vi "autonomous hard code.vi"   [LabVIEW 2012]
uses:
  <vilib>/Rock Robotics/WPI/Solenoid/WPI_SolenoidValue.ctl
  <vilib>/Rock Robotics/WPI/Solenoid/WPI_SolenoidSetEnum.vi
types:
  T1 = typedef "WPI_SolenoidValue.ctl" = enum16{"Off", "On", "Forward", "Reverse"}
  T2 = typedef "WPI_MotorControlDeviceRef.ctl" = cluster{"DeviceStatus":errorcluster, "Type":enum16{"PWM", "CAN"}, "PWM":cluster{"Digital Module":T3, "PWM Channel":T4, "DeadBand":T5}, "CAN":cluster{"Device Number":u8, "Control Mode":T6, "Semaphore":T7, "Max Vout":dbl}, "Invert":bool, "TransformRef":T8, "InvTransformRef":T8}
  T3 = typedef "FPGA_TypedefDigitalModule.ctl" = enum16{"Digital Module 1", "Digital Module 2"}
  T4 = typedef "FPGA_DIOPWMChannel.ctl" = enum8{"PWM 1", "PWM 2", "PWM 3", "PWM 4", "PWM 5", "PWM 6", "PWM 7", "PWM 8", "PWM 9", "PWM 10", "Invalid"}
  T5 = typedef "WPI_PWMDeadband.ctl" = cluster{"Name":string, "maxPositivePwm":i32, "minPositivePwm":i32, "centerPwm":i32, "maxNegativePwm":i32, "minNegativePwm":i32, "angularRange":u16}
  T6 = typedef "WPI_CANJaguar_ControlMode.ctl" = enum8{"Percent VBus", "Current", "Speed", "Position", "Voltage"}
  T7 = typedef "Semaphore RefNum" = refnum<k1>
  T8 = typedef "WPI_PWMTransform_ConPane.ctl" = refnum<vi>
  T9 = typedef "WPI_AnalogChannelDevRef.ctl" = cluster{"DevStatus":errorcluster, "Analog Module":T10, "Analog Channel":T11}
  T10 = typedef "FPGA_TypedefAnalogModule.ctl" = enum16{"Analog Module 1", "Analog Module 2"}
  T11 = typedef "FPGA_AIChannel.ctl" = enum8{"AI 1", "AI 2", "AI 3", "AI 4", "AI 5", "AI 6", "AI 7", "AI 8", "Invalid"}
  T12 = typedef "WPI_SolenoidDevRef.ctl" = cluster{"DevStatus":errorcluster, "Solenoid Module":T13, "Forward Solenoid Channel":T14, "Reverse Solenoid Channel":T14}
  T13 = typedef "FPGA_TypedefSolenoidModule.ctl" = enum16{"Solenoid Module 1", "Solenoid Module 2"}
  T14 = typedef "WPI_SolenoidChannel.ctl" = enum8{"Solenoid 1", "Solenoid 2", "Solenoid 3", "Solenoid 4", "Solenoid 5", "Solenoid 6", "Solenoid 7", "Solenoid 8", "Invalid"}
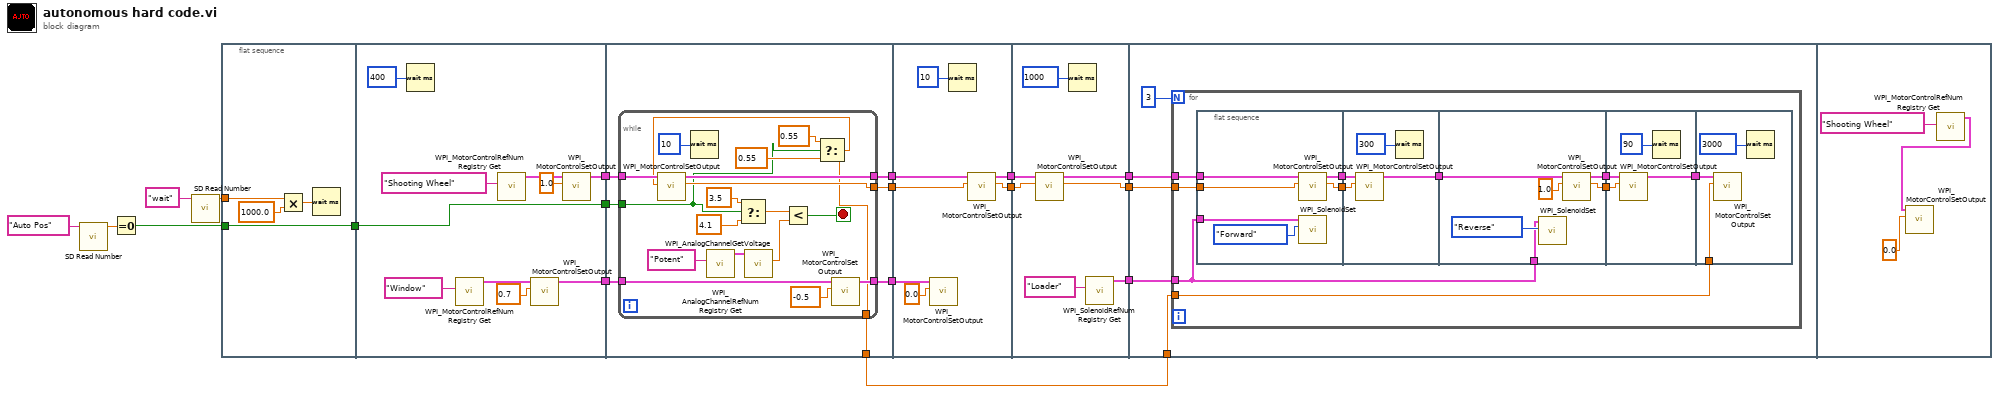
[diagram p0: block diagram]
diagram:
  n1 = call <vilib>:"SD Read Number.vi"("Name"="Auto Pos") -> ("Numeric"=w18:dbl)  [unwired: 8 in, 2 out]
  n2 = Equal To 0?(x=w18) -> (x = 0?=w14:bool)
  n3 = call <vilib>:"SD Read Number.vi"("Name"="wait") -> ("Numeric"=w15:dbl)  [unwired: 8 in, 2 out]
  n4 = flat-sequence {
    tunnel: w15 -> [w21]
    tunnel: [w19] -> w13
    tunnel: w14 -> [w19]
    tunnel: w13 -> [w27]
    tunnel: [w27] -> w12
    tunnel: [w29] -> w11
    tunnel: [w24] -> w6
    tunnel: w12 -> [w38]
    tunnel: w11 -> [w39]
    tunnel: [w37] -> w10
    tunnel: [w36] -> w9
    tunnel: w6 -> [w35]
    tunnel: [w34] -> w5
    tunnel: [w33] -> w1
    tunnel: w10 -> [w63]
    tunnel: w9 -> [w61]
    tunnel: [w60] -> w8
    tunnel: w5 -> [w59]
    tunnel: [w58] -> w4
    tunnel: w8 -> [w71]
    tunnel: [w69] -> w7
    tunnel: w4 -> [w68]
    tunnel: [w67] -> w3
    tunnel: [w65] -> w2
    tunnel: w7 -> [w76]
    tunnel: w3 -> [w72]
    tunnel: w1 -> [w75]
    tunnel: w2 -> [w73]
    frame #0 {
      n5 = Multiply(x=w21, y=1000.0) -> (x*y=w20:dbl)
      n6 = Wait (ms)(milliseconds to wait=w20) -> ()  [unwired: 1 out]
    }
    frame #1 {
      n7 = Wait (ms)(milliseconds to wait=u32 400) -> ()  [unwired: 1 out]
      n8 = call <vilib>:"WPI_MotorControlRefNum Registry Get.vi"("refnum name"="Window") -> ("MotorControlDevRef"=w32:T2)  [unwired: 9 in, 1 out]
      n9 = call <vilib>:"WPI_MotorControlRefNum Registry Get.vi"("refnum name"="Shooting Wheel") -> ("MotorControlDevRef"=w25:T2)  [unwired: 9 in, 1 out]
      n10 = call <vilib>:"WPI_MotorControlSetOutput.vi"("Output"=0.7, "MotorControlDevRef"=w32) -> ("MotorControlDevRef"=w29:T2)  [unwired: 7 in, 2 out]
      n11 = call <vilib>:"WPI_MotorControlSetOutput.vi"("Output"=1.0, "MotorControlDevRef"=w25) -> ("MotorControlDevRef"=w24:T2)  [unwired: 7 in, 2 out]
    }
    frame #2 {
      n12 = while {
        tunnel: w39 -> [w57]
        tunnel: w38 -> [w42]
        tunnel: [w48] -> w37
        tunnel: [w47] -> w36
        tunnel: w35 -> [w46]
        tunnel: [w45] -> w34
        tunnel: [w40] -> w33
        stop <- w50 stop-if-true
        n13 = Wait (ms)(milliseconds to wait=u32 10) -> ()  [unwired: 1 out]
        n14 = call <vilib>:"WPI_AnalogChannelRefNum Registry Get.vi"("refnum name"="Potent") -> ("AIDeviceRef"=w55:T9)  [unwired: 9 in, 1 out]
        n15 = Select(t=3.5, s=w42, f=4.1) -> (s? t:f=w53:dbl)
        n16 = call <vilib>:"WPI_AnalogChannelGetVoltage.vi"("AIDeviceRef"=w55) -> ("Voltage"=w54:dbl)  [unwired: 8 in, 2 out]
        n17 = Less?(x=w53, y=w54) -> (x < y?=w50:bool)
        n18 = Select(t=0.55, s=w42, f=0.55) -> (s? t:f=w40:dbl)
        n19 = call <vilib>:"WPI_MotorControlSetOutput.vi"("Output"=w40, "MotorControlDevRef"=w46) -> ("Motor Output"=w47:dbl, "MotorControlDevRef"=w45:T2)  [unwired: 7 in, 1 out]
        n20 = call <vilib>:"WPI_MotorControlSetOutput.vi"("Output"=-0.5 ("t"), "MotorControlDevRef"=w57) -> ("MotorControlDevRef"=w48:T2)  [unwired: 7 in, 2 out]
      }
    }
    frame #3 {
      n21 = call <vilib>:"WPI_MotorControlSetOutput.vi"("Output"=0.0, "MotorControlDevRef"=w63) -> ()  [unwired: 7 in, 3 out]
      n22 = Wait (ms)(milliseconds to wait=u32 10) -> ()  [unwired: 1 out]
      n23 = call <vilib>:"WPI_MotorControlSetOutput.vi"("Output"=w61, "MotorControlDevRef"=w59) -> ("Motor Output"=w60:dbl, "MotorControlDevRef"=w58:T2)  [unwired: 7 in, 1 out]
    }
    frame #4 {
      n24 = call <vilib>:"WPI_MotorControlSetOutput.vi"("Output"=w71, "MotorControlDevRef"=w68) -> ("Motor Output"=w69:dbl, "MotorControlDevRef"=w67:T2)  [unwired: 7 in, 1 out]
      n25 = Wait (ms)(milliseconds to wait=u32 1000) -> ()  [unwired: 1 out]
      n26 = call <vilib>:"WPI_SolenoidRefNum Registry Get.vi"("refnum name"="Loader") -> ("SolenoidDevRef"=w65:T12)  [unwired: 9 in, 1 out]
    }
    frame #5 {
      n27 = for {
        N: 3 -> [_]
        tunnel: w76 -> [w86]
        tunnel: w72 -> [w83]
        tunnel: w75 -> [w79]
        tunnel: w73 -> [w77]
        n28 = flat-sequence {
          tunnel: w86 -> [w91]
          tunnel: [w90] -> w85
          tunnel: w83 -> [w89]
          tunnel: [w88] -> w82
          tunnel: w77 -> [w87]
          tunnel: w85 -> [w95]
          tunnel: w82 -> [w94]
          tunnel: [w93] -> w81
          tunnel: [w100] -> w84
          tunnel: w81 -> [w99]
          tunnel: [w98] -> w80
          tunnel: w77 -> [w97]
          tunnel: w84 -> [w105]
          tunnel: w80 -> [w104]
          tunnel: [w103] -> w78
          tunnel: w79 -> [w109]
          tunnel: w78 -> [w108]
          frame #0 {
            n29 = call <vilib>:"WPI_MotorControlSetOutput.vi"("Output"=w91, "MotorControlDevRef"=w89) -> ("Motor Output"=w90:dbl, "MotorControlDevRef"=w88:T2)  [unwired: 7 in, 1 out]
            n30 = call-poly <vilib>:"WPI_SolenoidSet.vi"("Value"=WPI_SolenoidValue."Forward", "SolenoidDevRef"=w87) -> ()  [unwired: 8 in, 2 out]
          }
          frame #1 {
            n31 = call <vilib>:"WPI_MotorControlSetOutput.vi"("Output"=w95, "MotorControlDevRef"=w94) -> ("MotorControlDevRef"=w93:T2)  [unwired: 7 in, 2 out]
            n32 = Wait (ms)(milliseconds to wait=u32 300) -> ()  [unwired: 1 out]
          }
          frame #2 {
            n33 = call-poly <vilib>:"WPI_SolenoidSet.vi"("Value"=WPI_SolenoidValue."Reverse", "SolenoidDevRef"=w97) -> ()  [unwired: 8 in, 2 out]
            n34 = call <vilib>:"WPI_MotorControlSetOutput.vi"("Output"=1.0, "MotorControlDevRef"=w99) -> ("Motor Output"=w100:dbl, "MotorControlDevRef"=w98:T2)  [unwired: 7 in, 1 out]
          }
          frame #3 {
            n35 = call <vilib>:"WPI_MotorControlSetOutput.vi"("Output"=w105, "MotorControlDevRef"=w104) -> ("MotorControlDevRef"=w103:T2)  [unwired: 7 in, 2 out]
            n36 = Wait (ms)(milliseconds to wait=u32 90) -> ()  [unwired: 1 out]
          }
          frame #4 {
            n37 = call <vilib>:"WPI_MotorControlSetOutput.vi"("Output"=w109, "MotorControlDevRef"=w108) -> ()  [unwired: 7 in, 3 out]
            n38 = Wait (ms)(milliseconds to wait=u32 3000) -> ()  [unwired: 1 out]
          }
        }
      }
    }
    frame #6 {
      n39 = call <vilib>:"WPI_MotorControlRefNum Registry Get.vi"("refnum name"="Shooting Wheel") -> ("MotorControlDevRef"=w110:T2)  [unwired: 9 in, 1 out]
      n40 = call <vilib>:"WPI_MotorControlSetOutput.vi"("Output"=0.0, "MotorControlDevRef"=w110) -> ()  [unwired: 7 in, 3 out]
    }
  }
